vi "Init.vi"(8 "error in (no error)":errorcluster, 10 "Channel":i16, 11 "TrialBasedExperiment in":refnum<class "WNOriDiscExperiment.lvclass">) -> (0 "error out":errorcluster, 3 "TrialBasedExperiment out":refnum<class "WNOriDiscExperiment.lvclass">)   [LabVIEW 2011, in "WNOriDiscExperiment.lvclass"]
uses:
  WNOriDiscExperiment.lvclass
  TwoAfcEye/TwoAfcEye.lvclass
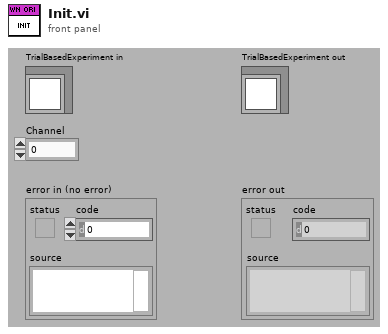
[diagram p1: front panel]
types:
  T1 = cluster{"Intertrial":dbl, "AcquireFixation":dbl, "HoldFixation":dbl, "DelayPeriod":dbl, "ResponsePeriod":dbl}
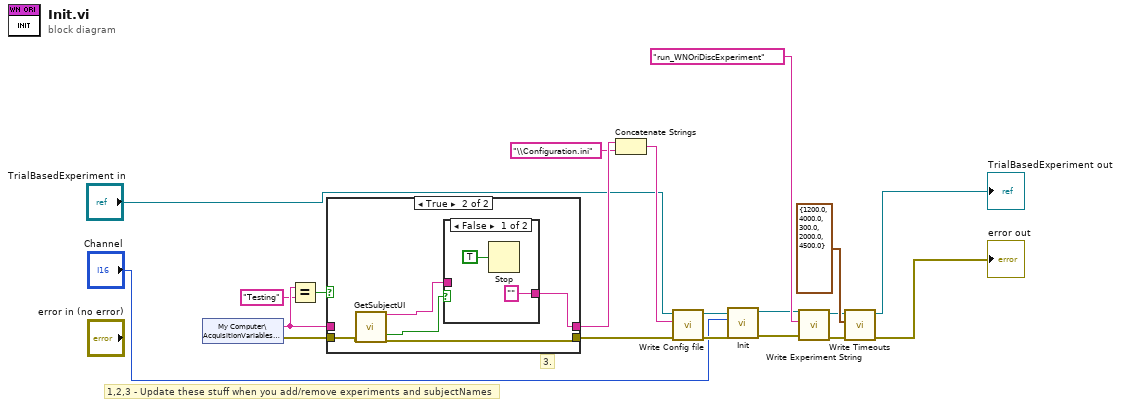
[diagram p0: block diagram]
diagram:
  # "1,2,3 - Update these stuff when you add/remove experiments and subjectNames"
  # "3."
  n1 = shared-variable "My Computer\\AcquisitionVariables.lvlib\\Subject"() -> (w17:string, error out=w18:errorcluster)  [unwired: 1 in]
  n2 = Equal?(x=w17, y="Testing") -> (x = y?=w15:bool)
  n3 = case shown="True" w15 {
    tunnel: [w22 w27] -> w20
    tunnel: w17 -> [w22 _]
    tunnel: w18 -> [w21 w23]
    tunnel: [w21 w24] -> w19
    frame False {
    }
    frame True {
      n4 = call "GetSubjectUI.vi"("error in (no error)"=w23) -> ("subjectSelected"=w26:string, "OK"=w25:bool, "error out"=w24:errorcluster)  [unwired: 16 in]
      n5 = case shown="False" w25 {
        tunnel: w26 -> [_ w30]
        tunnel: ["" ("subjectSelected") w30] -> w27
        frame False {
          n6 = Stop(stop? (T)=TRUE) -> ()
        }
        frame True {
        }
      }
    }
  }
  n7 = Concatenate Strings(w20, "\\Configuration.ini") -> (w13:string)
  n8 = call-dynamic "Write Config file.vi"("error in (no error)"=w19, "Config file"=w13, "TrialBasedExperiment in"="TrialBasedExperiment in") -> ("error out"=w6:errorcluster, "TrialBasedExperiment out"=w7:refnum<class "WNOriDiscExperiment.lvclass">)  [unwired: 7 in]
  n9 = call-parent "Init.vi"("error in (no error)"=w6, "Channel"="Channel", "TrialBasedExperiment in"=w7) -> ("error out"=w4:errorcluster, "TrialBasedExperiment out"=w5:refnum<class "WNOriDiscExperiment.lvclass">)  [unwired: 7 in]
  n10 = call-dynamic "Write Experiment String.vi"("error in (no error)"=w4, "Experiment String"="run_WNOriDiscExperiment" ("string"), "TrialBasedExperiment in"=w5) -> ("error out"=w10:errorcluster, "TrialBasedExperiment out"=w9:refnum<class "WNOriDiscExperiment.lvclass">)  [unwired: 7 in]
  n11 = call-dynamic "Write Timeouts.vi"("error in (no error)"=w10, "Timeouts"=T1 {"Intertrial"=1200.0, "AcquireFixation"=4000.0, "HoldFixation"=300.0, "DelayPeriod"=2000.0, "ResponsePeriod"=4500.0}, "TrialBasedExperiment in"=w9) -> ("error out"=→"error out":errorcluster, "TrialBasedExperiment out"=→"TrialBasedExperiment out":refnum<class "WNOriDiscExperiment.lvclass">)  [unwired: 7 in]
